vi "Destroy.vi"(0 "reference in":refnum<class "Iterator.lvclass">, 5 "error in (no error)":errorcluster) -> (14 "reference out":refnum<class "Iterator.lvclass">, 19 "error out":errorcluster)   [LabVIEW 2015, in "Iterator.lvclass"]
uses:
  Iterator.lvclass
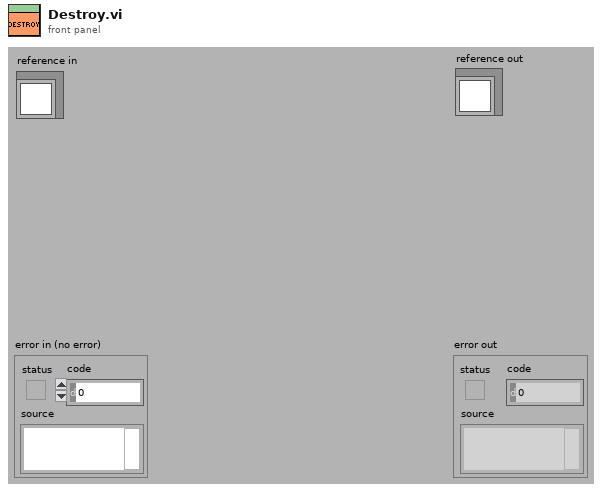
[diagram p1: front panel]
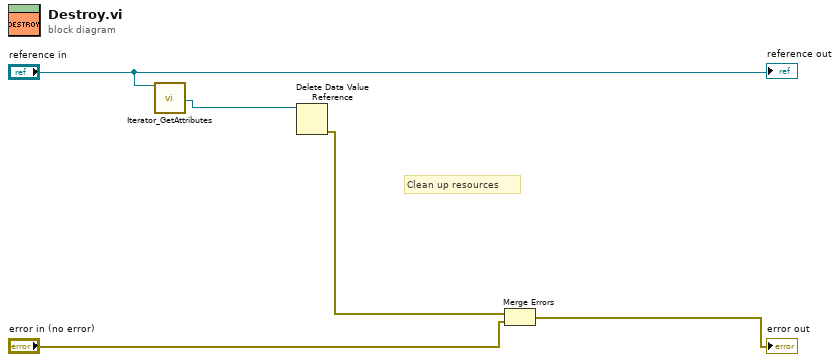
[diagram p0: block diagram]
diagram:
  # "Clean up resources"
  n1 = call "Iterator_GetAttributes.vi"("reference in"="reference in") -> ("DataRef"=w4:refnum<data-value>)  [unwired: 15 in, 3 out]
  n2 = Delete Data Value Reference(data value reference=w4) -> (error out=w3:errorcluster)  [unwired: 1 in, 1 out]
  n3 = Merge Errors(w3, "error in (no error)") -> (→"error out":errorcluster)
  "reference out" <- "reference in"
